vi "JSON to LVObject - Error Serialization Binder - Returns Error.vi"() -> ()   [LabVIEW 2017, in "Generic Object Serializer Tests.lvlib" / "Serialization Binder.lvlib"]
uses:
  Serialization Binder.lvlib
  Generic Object Serializer/Generic Object Serializer.lvclass
  Error Serialization Binder/Error Serialization Binder.lvclass
  C:/Users/de200256/Code/logmanoriginal/jsontext-object-serialization/Serialization Binder/Serialization Binder.lvclass
  Generic Object Serializer/Type Name Handling.ctl
  Generic Object Serializer/Generic Object Serializer.lvclass/Generic Object Serializer.ctl
  Generic Object Serializer/Write Serialization Binder.vi
  Generic Object Serializer/Write Type Name Handling.vi
  <vilib>/addons/_JKI Toolkits/Caraya/classes/Test/Test.lvclass
  <vilib>/addons/_JKI Toolkits/Caraya/classes/Assert/Assert.lvclass
panel:
  out "error out":errorcluster
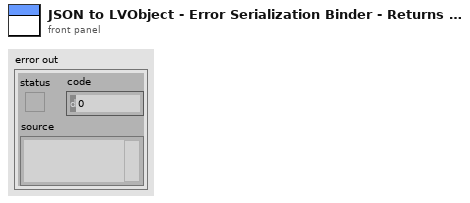
[diagram p1: front panel]
types:
  T1 = typedef "Generic Object Serializer.lvclass/Type Name Handling.ctl" = enum16{"None", "Inline"}
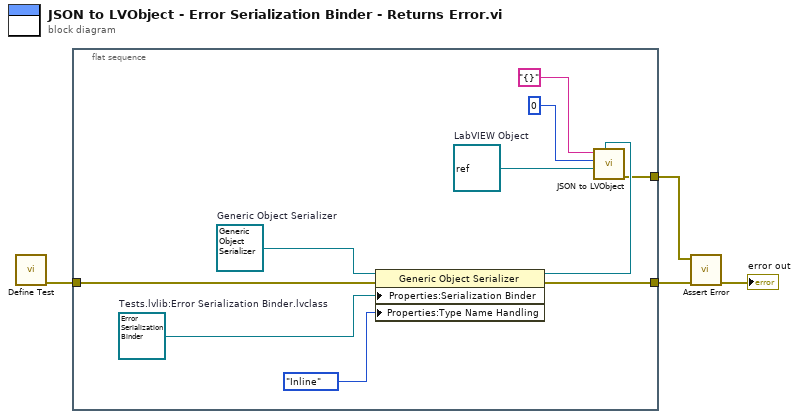
[diagram p0: block diagram]
diagram:
  n1 = call <vilib>:"Define Test.vi"() -> ("error out"=w4:errorcluster)  [unwired: 11 in]
  n2 = flat-sequence {
    tunnel: [w9] -> w3
    tunnel: w4 -> [w13]
    tunnel: [w8] -> w1
    frame #0 {
      w11 = refnum<class> refnum  # LabVIEW Object
      w12 = refnum<class "Error Serialization Binder.lvclass"> refnum  # Tests.lvlib:Error Serialization Binder.lvclass
      w14 = refnum<class "Generic Object Serializer.lvclass"> refnum  # Generic Object Serializer
      n3 = property class="Generic Object Serializer"(reference=w14, error in=w13, "Properties:Serialization Binder"=w12, "Properties:Type Name Handling"=Type_Name_Handling."Inline" ("Type Name Handling")) -> (reference out=w10:refnum<class "Generic Object Serializer.lvclass">, error out=w9:errorcluster)
      n4 = call-dynamic "JSON to LVObject.vi"("LVClass Serializer"=w10, "Object Type"=w11, "Offset"=0, "JSON"="{}") -> ("error out"=w8:errorcluster)  [unwired: 6 in, 1 out]
    }
  }
  n5 = call <vilib>:"Assert Error.vi"("error in (no error)"=w3, "Error?"=w1) -> ("error out"=→"error out":errorcluster)  [unwired: 9 in]
